vi "Get Instrument.vi"(8 "error in (no error)":errorcluster, 11 "Virt Instr Base in":refnum<class "Virt Instr Host.lvclass">) -> (0 "error out":errorcluster, 2 "HAL GOOP4.lvlib:Instrument":refnum<class "Instrument.lvclass">, 3 "Virt Instr Base out":refnum<class "Virt Instr Host.lvclass">)   [LabVIEW 2023, in "HAL GOOP4.lvlib" / "Virt Instr Host.lvclass"]
uses:
  Virt Instr Host.lvclass
  Instrument/Instrument.lvclass
  Virt Instr Host.lvclass/Virt Instr Host.ctl
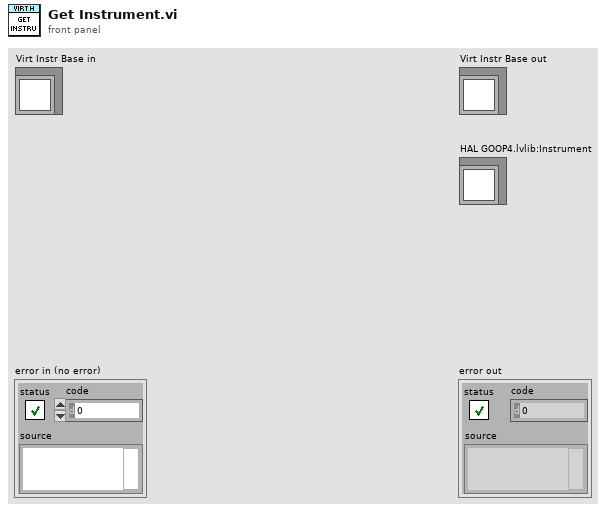
[diagram p1: front panel]
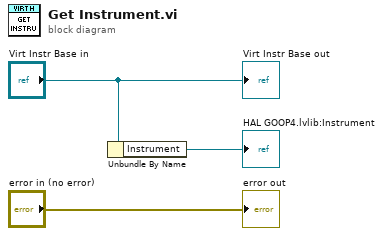
[diagram p0: block diagram]
diagram:
  n1 = Unbundle By Name("Virt Instr Base in") -> ("Instrument"=→"HAL GOOP4.lvlib:Instrument":refnum<class "Instrument.lvclass">)
  "error out" <- "error in (no error)"
  "Virt Instr Base out" <- "Virt Instr Base in"
